vi "Set Property.vi"(10 "Ctl Ref":refnum<vi>, 11 "UIP In":refnum<class "SizeUIP.lvclass">) -> (0 "Error Out":errorcluster, 3 "UIP Out":refnum<class "SizeUIP.lvclass">)   [LabVIEW 2015, in "SizeUIP.lvclass"]
doc: "Modify this method to implement functionality for applying the UIP data to the property from VI Server Control."
uses:
  SizeUIP.lvclass
  SizeUIP.lvclass/SizeUIP.ctl
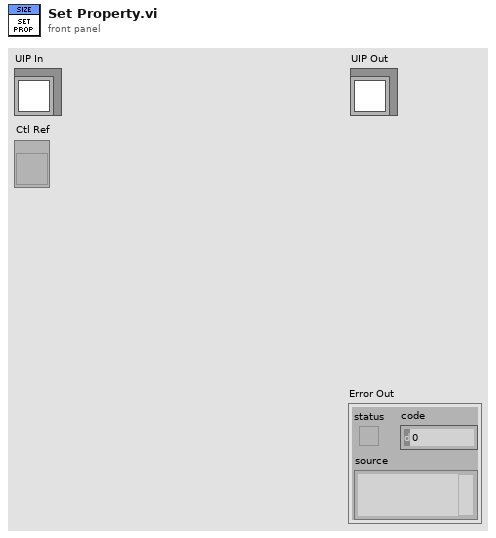
[diagram p1: front panel]
types:
  T1 = typedef "LVBoundsTypeDef.ctl" = cluster{"Width":u32, "Height":u32}
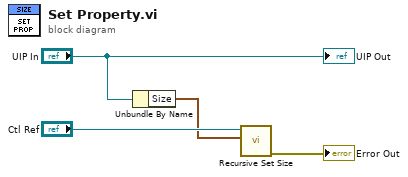
[diagram p0: block diagram]
diagram:
  n1 = Unbundle By Name("UIP In") -> ("Size"=w2:T1)
  n2 = call "Recursive Set Size.vi"("Size"=w2, "Control"="Ctl Ref") -> ("error out"=→"Error Out":errorcluster)  [unwired: 9 in]
  "UIP Out" <- "UIP In"
